vi "Measure.vi"(8 "error in (no error)":errorcluster, 11 "SimDaq in":refnum<class "SimDaq.lvclass">) -> (0 "error out":errorcluster, 3 "SimDaq out":refnum<class "SimDaq.lvclass">)   [LabVIEW 2020, in "SimDaq.lvlib" / "SimDaq.lvclass"]
uses:
  SimDaq.lvclass
  <vilib>/measure/NI_MABase.lvlib
  <vilib>/ActorFramework/Actor/Actor.lvclass
  TransferData Messages/ReceiveWaveform Msg/ReceiveWaveform Msg.lvclass
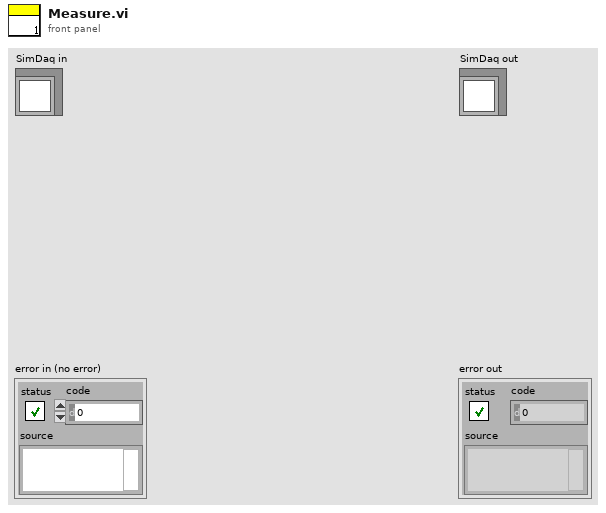
[diagram p1: front panel]
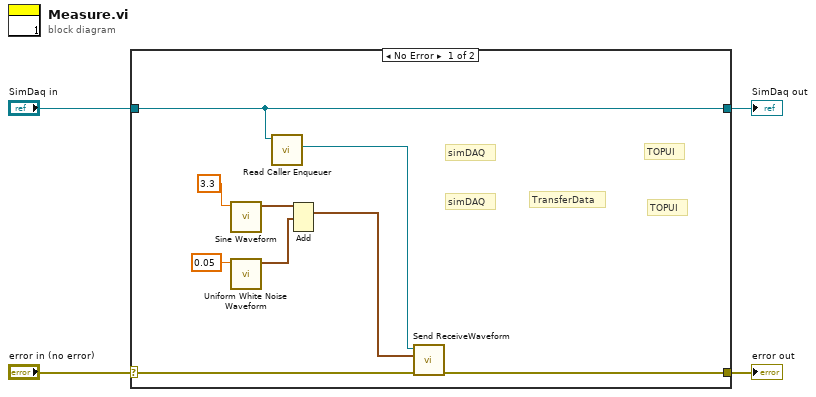
[diagram p0: block diagram]
diagram:
  n1 = case shown="No Error" "error in (no error)" {
    selector: "error in (no error)" -> [w8 w15]
    tunnel: [w7 w15] -> w3
    tunnel: [w10 w14] -> w1
    tunnel: "SimDaq in" -> [w10 w14]
    frame No Error {
      # "TOPUI"
      # "simDAQ"
      # "TOPUI"
      # "TransferData"
      # "simDAQ"
      n2 = call <vilib>:"Sine Waveform.vi"("frequency"=3.3) -> ("signal out"=w13:waveform(dbl))  [unwired: 9 in, 1 out]
      n3 = call <vilib>:"Uniform White Noise Waveform.vi"("amplitude"=0.05) -> ("signal out"=w12:waveform(dbl))  [unwired: 9 in, 1 out]
      n4 = call <vilib>:"Read Caller Enqueuer.vi"("Actor"=w10) -> ("Caller Enqueuer"=w6:refnum<class "Message Enqueuer.lvclass">)  [unwired: 10 in]
      n5 = Add(1:w12, 2:w13) -> (0:w5:waveform(dbl))  [unwired: 1 in, 1 out]
      n6 = call "Send ReceiveWaveform.vi"("error in (no error)"=w8, "Waveform"=w5, "Message Enqueuer"=w6) -> ("error out"=w7:errorcluster)  [unwired: 7 in, 1 out]
    }
    frame Error {
    }
  }
  "error out" <- w3
  "SimDaq out" <- w1
